vi "GetProperties.vi"(8 "error in":errorcluster, 11 "Ring in":refnum<class "Ring.lvclass">) -> (0 "error out":errorcluster, 3 "Ring out":refnum<class "Ring.lvclass">)   [LabVIEW 2014, in "Raspberry Pi Compatible Compiler for LabVIEW.lvlib" / "Ring.lvclass"]
uses:
  Ring.lvclass
  Ring.lvclass/Ring.ctl
  NamedNumeric/NamedNumeric.lvclass
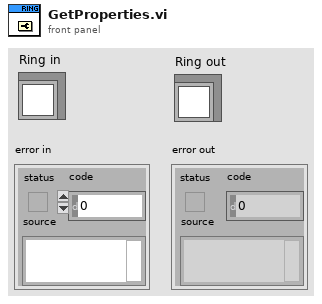
[diagram p1: front panel]
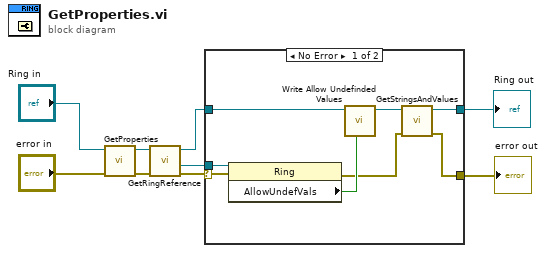
[diagram p0: block diagram]
diagram:
  n1 = call-parent "GetProperties.vi"("error in"="error in", "NamedNumeric in"="Ring in") -> ("error out"=w6:errorcluster, "NamedNumeric out"=w7:refnum<class "Ring.lvclass">)  [unwired: 8 in]
  n2 = call "GetRingReference.vi"("error in"=w6, "Ring in"=w7) -> ("error out"=w5:errorcluster, "Ring reference"=w4:refnum<vi>, "Ring out"=w3:refnum<class "Ring.lvclass">)  [unwired: 7 in]
  n3 = case shown="No Error" w5 {
    selector: w5 -> [w17 w18]
    tunnel: w4 -> [w16 _]
    tunnel: w3 -> [w14 w19]
    tunnel: [w10 w18] -> w1
    tunnel: [w12 w19] -> w2
    frame No Error {
      n4 = property class="Ring"(reference=w16, error in=w17) -> (error out=w11:errorcluster, "AllowUndefVals"=w15:bool)  [unwired: 1 out]
      n5 = call "Write Allow Undefinded Values.vi"("Allow Undefinded Values"=w15, "Ring in"=w14) -> ("Ring out"=w13:refnum<class "Ring.lvclass">)  [unwired: 7 in]
      n6 = call "GetStringsAndValues.vi"("error in"=w11, "Ring in"=w13) -> ("error out"=w10:errorcluster, "Ring out"=w12:refnum<class "Ring.lvclass">)  [unwired: 8 in]
    }
    frame Error {
    }
  }
  "error out" <- w1
  "Ring out" <- w2
